vi "Joystick Set Outputs.vi"(7 "color":u32(colorbox), 8 "error in (no error)":errorcluster, 9 "trigger rumble":cluster{"Left":sgl, "Right":sgl}, 10 "rumble":cluster{"Left":sgl, "Right":sgl}, 11 "Joystick":T1) -> (0 "error out":errorcluster, 3 "Joystick":T1)   [LabVIEW 2026, in "MrcLib.lvlib"]
doc: "Updates rumble and driven outputs for a USB joystick device that you specify."
uses:
  MrcLib.lvlib
  <vilib>/Rock Robotics/WPI/Joystick/WPI_JoystickDeviceEnum.ctl
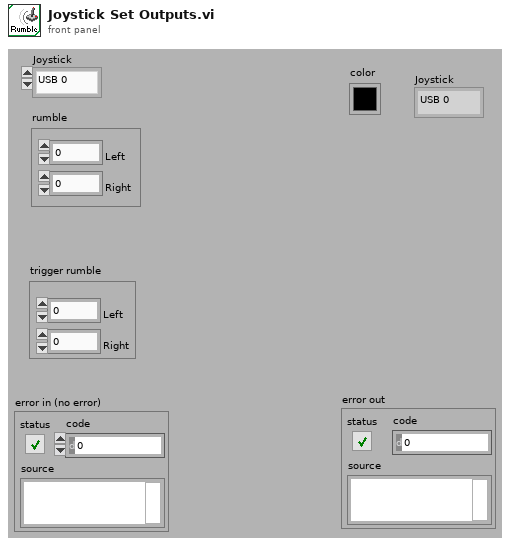
[diagram p1: front panel]
types:
  T1 = typedef "WPI_JoystickDeviceEnum.ctl" = enum16{"USB 0", "USB 1", "USB 2", "USB 3", "USB 4", "USB 5"}
  T2 = cluster{"R":u8, "G":u8, "B":u8, "B":u8, u16, u16, u16, u16}
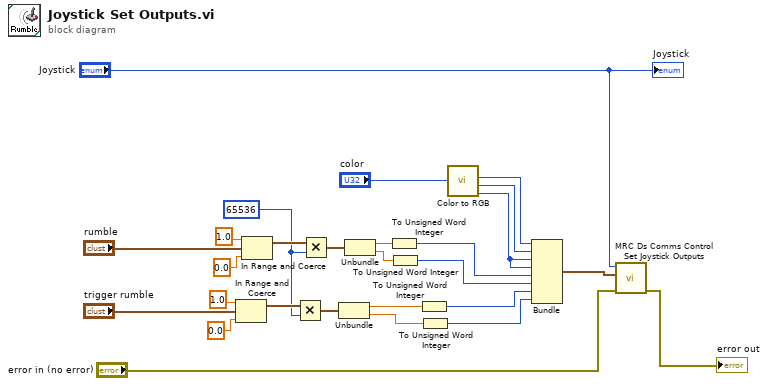
[diagram p0: block diagram]
diagram:
  w6 = 65536
  n1 = In Range and Coerce(upper limit=1.0, x="trigger rumble", lower limit=0.0) -> (coerced(x)=w15:cluster{"Left":sgl, "Right":sgl})  [unwired: 1 out]
  n2 = In Range and Coerce(upper limit=1.0, x="rumble", lower limit=0.0) -> (coerced(x)=w8:cluster{"Left":sgl, "Right":sgl})  [unwired: 1 out]
  n3 = Multiply(x=w15, y=w6) -> (x*y=w14:cluster{"Left":sgl, "Right":sgl})
  n4 = Multiply(x=w8, y=w6) -> (x*y=w9:cluster{"Left":sgl, "Right":sgl})
  n5 = Unbundle(w14) -> ("Left"=w12:sgl, "Right"=w13:sgl)
  n6 = Unbundle(w9) -> ("Left"=w4:sgl, "Right"=w3:sgl)
  n7 = To Unsigned Word Integer(number=w4) -> (unsigned 16bit integer=w22:u16)
  n8 = To Unsigned Word Integer(number=w3) -> (unsigned 16bit integer=w21:u16)
  n9 = To Unsigned Word Integer(number=w12) -> (unsigned 16bit integer=w20:u16)
  n10 = To Unsigned Word Integer(number=w13) -> (unsigned 16bit integer=w19:u16)
  n11 = call <vilib>:"Color to RGB.vi"("Color"="color") -> ("R"=w24:u8, "G"=w23:u8, "B"=w18:u8)  [unwired: 1 out]
  n12 = Bundle("R"=w24, "G"=w23, "B"=w18, "B"=w18, w22, w21, w20, w19) -> (w27:T2)  [unwired: 1 in]
  n13 = call "MRC Ds Comms Control Set Joystick Outputs.vi"("error in (no error)"="error in (no error)", "outputs"=w27, "stickIndex"="Joystick") -> ("error out"=→"error out":errorcluster)  [unwired: 8 in]
  "Joystick" <- "Joystick"
